vi "transfer1Dto2DArray.vi"(10 "Array in":i32[](array[numeric]), 11 "Width":u16) -> (3 "Array out":i32[][](array[numeric]))   [LabVIEW 2016]
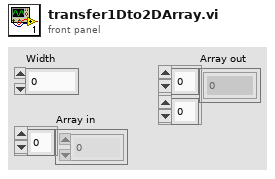
[diagram p1: front panel]
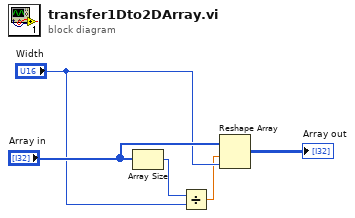
[diagram p0: block diagram]
diagram:
  n1 = Array Size(array="Array in") -> (size(s)=w1:i32)
  n2 = Divide(x=w1, y="Width") -> (x/y=w2:dbl)
  n3 = Reshape Array("Array in", w2, "Width") -> (→"Array out":i32[][])
